vi "goBallTargetDirection.vi"(4 "NewParameters":T2={"PenaltyDistance"=0.0, "DistanceAttackerToBackBall"=0.0, "Division"=enum."Div B", "DistanceToAvoidyEnemyRobot"=0.0, "BallPlacementDistance"=900.0, "DisatanceBehindBallToStealBall"=0.0, "MaxDistanceToPositionKickoff"=2000.0, "BlockEnemyTarget"=FALSE, "MaxStopVAng"=1.0, "DistanceMarkerToEnemy"=0.0, "IgnoreDribblerContact"=FALSE, "DistanceToBeginEnemyPosession"=200.0, "GoToBallWhenEnemyNotMoving"=TRUE, "EnemyDistanceToReduceVelocity"=500.0, "TurnOnEnemyDistanceToReduceVelocity"=TRUE, "EnemyDistanceToShootOutBall"=500.0, "DefenseKickBall"=TRUE, "MoreKickToGoal? (0-0.3)"=0.0, "ChipKickInEnemyField"=TRUE, "ShootOutRobotId"=0.0, "FieldLenghtDenominatorInShootOut"=0.0, "AdjustPositionInBallPlacement"=FALSE, "PowerGodPass"=0.0, "VelocityAbortEnemyPos"=0.0, "MaxDistToBeginPass"=500.0, "MinDistToBeginPass"=150.0, "VelocityInDirects"=0.3, "BadDribblerIDs"=[], "NewKickToDistanceAroundBall"=300.0, "PowerAvoidColisionMarker"=0.5, "DistanceToAvoidColisionMarker"=250.0, "AvoidBallKick"=0.0, "DistanceTryKick"=0.0, "SuicideKickDIstance"=0.0, "FirstKickAtck"=FALSE, "AdjustFirstKickDistance"=0.0, "FirstKickDefense"=FALSE, "AvoidAimLessKick"=0.0, "DistanceToAvoidyEnemyShootRobot "=0.0, "NumberOfMarkers"=3.0, "PotField"=TRUE, "PIDLateral"=FALSE, "MinDistanceFirstKickX"=0.0, "MinDistanceFirstKickY"=0.0, "FractionOfDistToTouchGround\nAfterChipKick"=0.8, "FractionOfKickxWhen\nComposedWithKickz"=0.0, "Style"=enum."Insanity", "MoveInTurnState"=TRUE, "DistFromEnemyToConsider\nMoveInTurnState"=0.0}, 6 "Target":dbl[](array[numeric]), 7 "state":T1, 8 "error in (no error)":errorcluster, 9 "BallRef":refnum<class "Ball.lvclass">, 10 "Robot":refnum<class "Robot.lvclass">, 11 "Utilities in":refnum<class "Utilities.lvclass">) -> (0 "error out":errorcluster, 1 "dest_y":dbl, 2 "dest_x":dbl, 3 "Utilities out":refnum<class "Utilities.lvclass">)   [LabVIEW 2020, in "Utilities.lvclass"]
uses:
  Utilities.lvclass
  Robot_class/Robot.lvclass
  C:/Users/anton/Desktop/RoboIME/IC/SSL_AI/Object_class/Object.lvclass
  Ball_class/Ball.lvclass
  Controls/NewParameters.ctl
  Style.ctl
  Robot_class/robotKickToStates.ctl
  Object_class/Object.lvclass/Object.ctl
  <vilib>/Analysis/_algsub.llb/Real Vector Norm.vi
  <vilib>/Analysis/baseanly.llb/Unit Vector (DBL).vi
  Object_class/Read position(x,y).vi
  <vilib>/Analysis/NI_AALBase.lvlib
  <vilib>/Analysis/NI_AALPro.lvlib
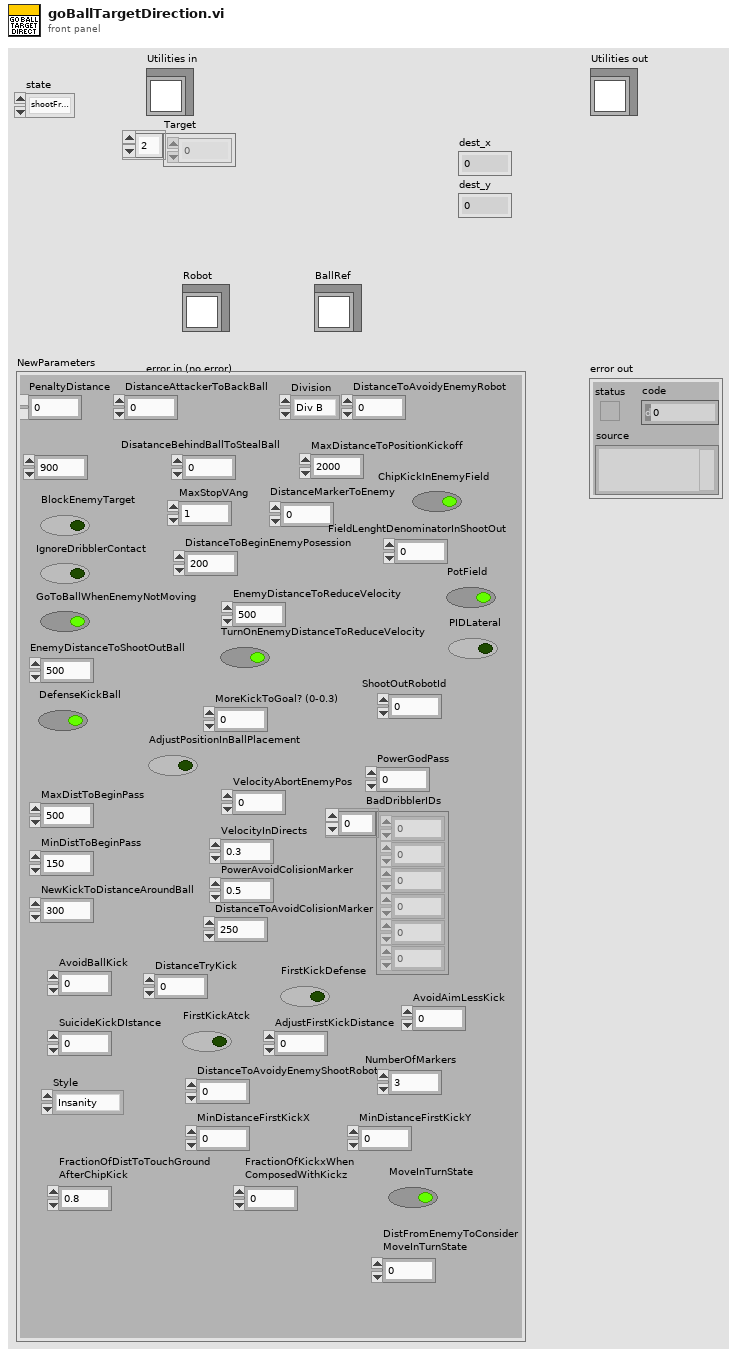
[diagram p1: front panel]
types:
  T1 = typedef "robotKickToStates.ctl" = enum16{"shootFromDirect", "avoidCollideBall", "goToBackBall", "none", "walk", "turn", "oldKickToShoot", "oldKickToGoToBackBall", "shoot"}
  T2 = typedef "NewParameters.ctl" = cluster{"PenaltyDistance":dbl, "DistanceAttackerToBackBall":dbl, "Division":enum16{"Div B", "Div A"}, "DistanceToAvoidyEnemyRobot":dbl, "BallPlacementDistance":dbl, "DisatanceBehindBallToStealBall":dbl, "MaxDistanceToPositionKickoff":dbl, "BlockEnemyTarget":bool, "MaxStopVAng":dbl, "DistanceMarkerToEnemy":dbl, "IgnoreDribblerContact":bool, "DistanceToBeginEnemyPosession":dbl, "GoToBallWhenEnemyNotMoving":bool, "EnemyDistanceToReduceVelocity":dbl, "TurnOnEnemyDistanceToReduceVelocity":bool, "EnemyDistanceToShootOutBall":dbl, "DefenseKickBall":bool, "MoreKickToGoal? (0-0.3)":dbl, "ChipKickInEnemyField":bool, "ShootOutRobotId":dbl, "FieldLenghtDenominatorInShootOut":dbl, "AdjustPositionInBallPlacement":bool, "PowerGodPass":dbl, "VelocityAbortEnemyPos":dbl, "MaxDistToBeginPass":dbl, "MinDistToBeginPass":dbl, "VelocityInDirects":dbl, "BadDribblerIDs":i32[], "NewKickToDistanceAroundBall":dbl, "PowerAvoidColisionMarker":dbl, "DistanceToAvoidColisionMarker":dbl, "AvoidBallKick":dbl, "DistanceTryKick":dbl, "SuicideKickDIstance":dbl, "FirstKickAtck":bool, "AdjustFirstKickDistance":dbl, "FirstKickDefense":bool, "AvoidAimLessKick":dbl, "DistanceToAvoidyEnemyShootRobot ":dbl, "NumberOfMarkers":dbl, "PotField":bool, "PIDLateral":bool, "MinDistanceFirstKickX":dbl, "MinDistanceFirstKickY":dbl, "FractionOfDistToTouchGround\nAfterChipKick":dbl, "FractionOfKickxWhen\nComposedWithKickz":dbl, "Style":T3, "MoveInTurnState":bool, "DistFromEnemyToConsider\nMoveInTurnState":dbl}
  T3 = typedef "Style.ctl" = enum16{"Insanity", "Offensive", "Defensive"}
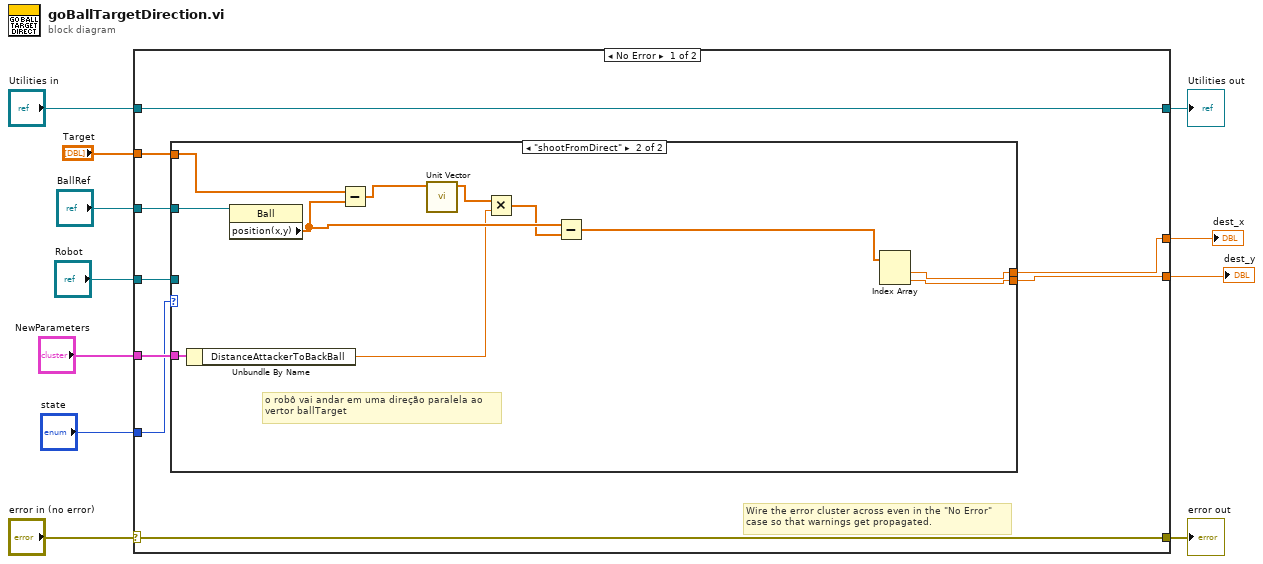
[diagram p0: block diagram]
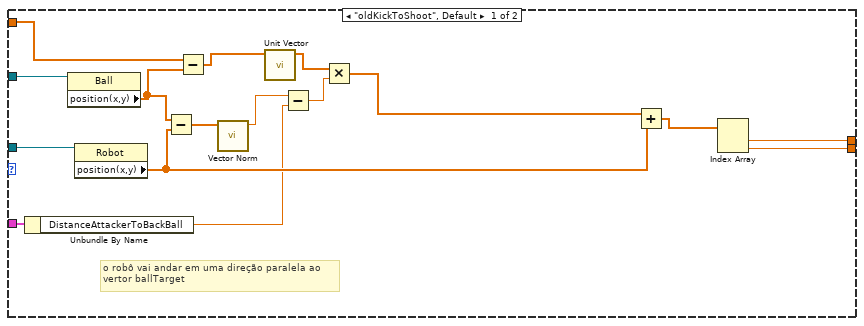
[diagram p2: hidden frame]
diagram:
  n1 = case shown="No Error" "error in (no error)" {
    selector: "error in (no error)" -> [w19 w49]
    tunnel: [w19 w49] -> w10
    tunnel: [w20 w48] -> w8
    tunnel: "Utilities in" -> [w20 w48]
    tunnel: [w14 _] -> w7
    tunnel: [w15 _] -> w6
    tunnel: "Robot" -> [w16 _]
    tunnel: "BallRef" -> [w18 _]
    tunnel: "Target" -> [w17 _]
    tunnel: "NewParameters" -> [w13 _]
    tunnel: "state" -> [w12 _]
    frame No Error {
      # "Wire the error cluster across even in the \"No Error\"\ncase so that warnings get propagated."
      n2 = case shown="\"shootFromDirect\"" w12 {
        tunnel: w18 -> [w36 w47]
        tunnel: w17 -> [w35 w46]
        tunnel: w16 -> [w33 _]
        tunnel: [w29 w38] -> w15
        tunnel: [w28 w37] -> w14
        tunnel: w13 -> [w24 w42]
        frame "oldKickToShoot", Default {
          # "o robô vai andar em uma direção paralela ao\nvertor ballTarget"
          n3 = Unbundle By Name(w24) -> ("DistanceAttackerToBackBall"=w22:dbl)
          n4 = property class="Ball"(reference=w36) -> ("position(x,y)"=w27:dbl[])  [unwired: 1 in, 2 out]
          n5 = property class="Robot"(reference=w33) -> ("position(x,y)"=w26:dbl[])  [unwired: 1 in, 2 out]
          n6 = Subtract(x=w27, y=w26) -> (x-y=w25:dbl[])
          n7 = Subtract(x=w35, y=w27) -> (x-y=w34:dbl[])
          n8 = call-poly <vilib>:"Vector Norm.vi"("Input Vector"=w25) -> ("norm"=w23:dbl)  [unwired: 9 in, 1 out]
          n9 = call-poly <vilib>:"Unit Vector.vi"("Input Vector"=w34) -> ("Unit Vector"=w32:dbl[])  [unwired: 8 in, 2 out]
          n10 = Subtract(x=w23, y=w22) -> (x-y=w21:dbl)
          n11 = Multiply(x=w32, y=w21) -> (x*y=w31:dbl[])
          n12 = Add(x=w31, y=w26) -> (x+y=w30:dbl[])
          n13 = Index Array(array=w30) -> (element #1=w29:dbl, element #2=w28:dbl)  [unwired: 2 in]
        }
        frame "shootFromDirect" {
          # "o robô vai andar em uma direção paralela ao\nvertor ballTarget"
          n14 = Unbundle By Name(w42) -> ("DistanceAttackerToBackBall"=w40:dbl)
          n15 = property class="Ball"(reference=w47) -> ("position(x,y)"=w43:dbl[])  [unwired: 1 in, 2 out]
          n16 = Subtract(x=w46, y=w43) -> (x-y=w45:dbl[])
          n17 = call-poly <vilib>:"Unit Vector.vi"("Input Vector"=w45) -> ("Unit Vector"=w44:dbl[])  [unwired: 8 in, 2 out]
          n18 = Multiply(x=w44, y=w40) -> (x*y=w41:dbl[])
          n19 = Subtract(x=w43, y=w41) -> (x-y=w39:dbl[])
          n20 = Index Array(array=w39) -> (element #1=w38:dbl, element #2=w37:dbl)  [unwired: 2 in]
        }
      }
    }
    frame Error {
    }
  }
  "error out" <- w10
  "Utilities out" <- w8
  "dest_x" <- w6
  "dest_y" <- w7
